vi "Stop_Spin.vi"(8 "error in (no error)":errorcluster, 11 "SpinCoater in":refnum<class "SpinCoater.lvclass">) -> (0 "error out":errorcluster, 3 "SpinCoater out":refnum<class "SpinCoater.lvclass">)   [LabVIEW 2020, in "SpinCoater.lvclass"]
uses:
  <instrlib>/Classes/SpinCoater/SpinCoater.lvclass
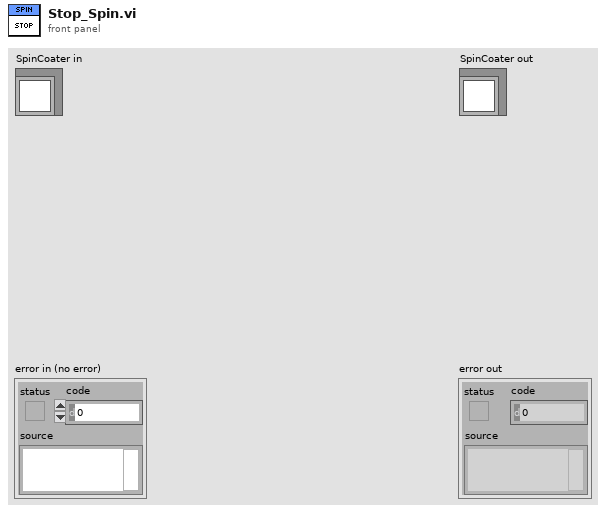
[diagram p1: front panel]
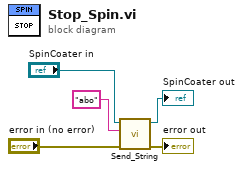
[diagram p0: block diagram]
diagram:
  n1 = call-dynamic "Send_String.vi"("error in (no error)"="error in (no error)", "String"="abo" ("write buffer"), "SpinCoater in"="SpinCoater in") -> ("error out"=→"error out":errorcluster, "SpinCoater out"=→"SpinCoater out":refnum<class "SpinCoater.lvclass">)  [unwired: 6 in, 1 out]
